vi "get_single_acq.vi"(8 "error in (no error)":errorcluster, 11 "dummy in":refnum<class "dummy.lvclass">) -> (0 "error out":errorcluster, 1 "trigger":bool[][](array[boolean]), 2 "raw data":i32[][][](array[numeric]), 3 "dummy out":refnum<class "dummy.lvclass">)   [LabVIEW 2019, in "dummy.lvlib" / "dummy.lvclass"]
uses:
  dummy.lvclass
  D:/github/TransientAbsorptionDAQ.lv/_camera/_camera.lvlibp/_cameraClass/_camera.lvclass
  _camera/_camera.lvlibp/_cameraClass/Read stage positions.vi
  _camera/_camera.lvlibp/_cameraClass/Read background.vi
  <vilib>/gmath/NI_Gmath.lvlib
  <vilib>/Analysis/NI_AALBase.lvlib
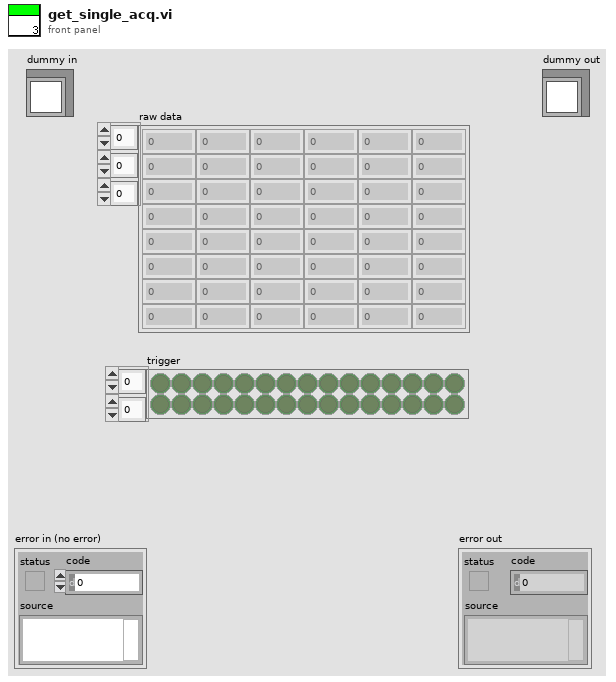
[diagram p1: front panel]
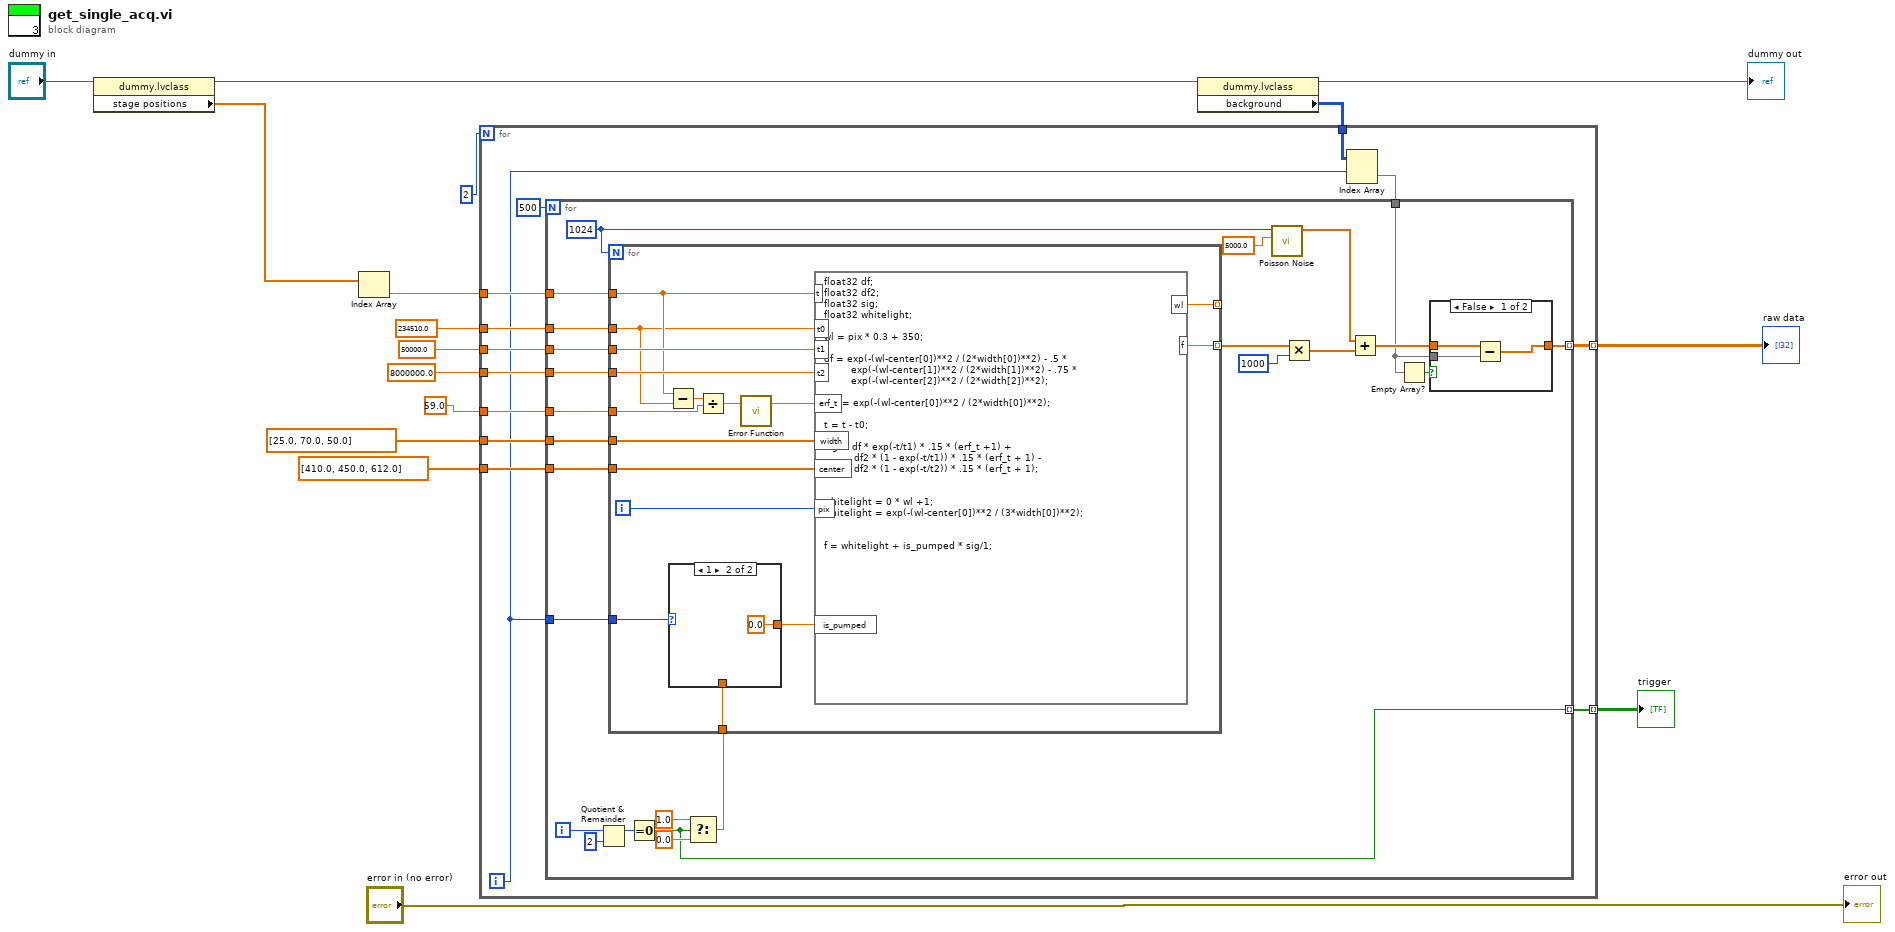
[diagram p0: block diagram]
diagram:
  n1 = property class="dummy.lvclass"(reference="dummy in") -> (reference out=w1:refnum<class "dummy.lvclass">, "stage positions"=w3:dbl[])  [unwired: 1 in, 1 out]
  n2 = Index Array(array=w3) -> (element=w5:dbl)  [unwired: 1 in]
  n3 = property class="dummy.lvclass"(reference=w1) -> (reference out=→"dummy out":refnum<class "dummy.lvclass">, "background"=w6:i32[][])  [unwired: 1 in, 1 out]
  n4 = for {
    N: 2 -> [_]
    tunnel: dbl[] [410.0, 450.0, 612.0] -> [w28]
    tunnel: dbl[] [25.0, 70.0, 50.0] -> [w27]
    tunnel: w5 -> [w26]
    tunnel: 234510.0 -> [w25]
    tunnel: 8000000.0 ("input variable") -> [w24]
    tunnel: 50000.0 ("input variable") -> [w23]
    tunnel: 59.0 ("y") -> [w22]
    tunnel: [w21] -> w9 mode=indexing
    tunnel: [w20] -> w8 mode=indexing
    tunnel: w6 -> [w19]
    i -> [w18]
    n5 = Index Array(array=w19, index (row)=w18) -> (element=w17:i32[])  [unwired: 1 in]
    n6 = for {
      N: 500 -> [_]
      tunnel: w28 -> [w54]
      tunnel: w27 -> [w53]
      tunnel: w26 -> [w52]
      tunnel: w25 -> [w51]
      tunnel: w24 -> [w50]
      tunnel: w23 -> [w49]
      tunnel: w22 -> [w48]
      tunnel: [w32] -> w21 mode=indexing
      tunnel: [w36] -> w20 mode=indexing
      tunnel: w18 -> [w35]
      tunnel: w17 -> [w30]
      i -> [w43]
      w40 = 1024
      n7 = Quotient & Remainder(x=w43, y=2) -> (x-y*floor(x/y)=w47:i32)  [unwired: 1 out]
      n8 = Equal To 0?(x=w47) -> (x = 0?=w36:bool)
      n9 = Select(t=1.0, s=w36, f=0.0) -> (s? t:f=w34:dbl)
      n10 = for {
        N: w40 -> [_]
        tunnel: w54 -> [w73]
        tunnel: w53 -> [w72]
        tunnel: w52 -> [w64]
        tunnel: w51 -> [w63]
        tunnel: w50 -> [w71]
        tunnel: w49 -> [w70]
        tunnel: w48 -> [w66]
        tunnel: [w62] -> w42 mode=indexing
        tunnel: [w65] -> _ mode=indexing
        tunnel: w35 -> [w61]
        tunnel: w34 -> [w59]
        i -> [w74]
        n11 = Subtract(x=w64, y=w63) -> (x-y=w68:dbl)
        n12 = case shown="1" w61 {
          tunnel: [w75 0.0 ("f")] -> w60
          tunnel: w59 -> [w75 _]
          frame 0, Default {
          }
          frame 1 {
          }
        }
        n13 = Divide(x=w68, y=w66) -> (x/y=w67:dbl)
        n14 = call <vilib>:"Error Function.vi"("x"=w67) -> ("erf(x)"=w69:dbl)  [unwired: 2 in]
        n15 = formula code="float32 df;\nfloat32 df2;\nfloat32 sig;\nfloat32 whitelight;\n\nwl = pix * 0.3 + 350;\n\ndf = exp(-(wl-center[0])**2 / (2*width[0])**2) - .5 *\n         exp(-(wl-center[1])**2 / (2*width[1])**2) - .75 * \n         exp(-(wl-center[2])**2 / (2*width[2])**2);\n\ndf2 = exp(-(wl-center[0])**2 / (2*width[0])**2);\n\nt = t - t0;\n\nsig = df * exp(-t/t1) * .15 * (erf_t +1) +\n          df2 * (1 - exp(-t/t1)) * .15 * (erf_t + 1) -\n          df2 * (1 - exp(-t/t2)) * .15 * (erf_t + 1);\n\n\nwhitelight = 0 * wl +1;\nwhitelight = exp(-(wl-center[0])**2 / (3*width[0])**2);\n\n\nf = whitelight + is_pumped * sig/1;"("pix"=w74, "center"=w73, "width"=w72, "t"=w64, "t0"=w63, "t1"=w70, "t2"=w71, "erf_t"=w69, "is_pumped"=w60) -> ("wl"=w65:dbl, "f"=w62:dbl)
      }
      n16 = call <vilib>:"Poisson Noise.vi"("mean"=5000.0, "samples"=w40) -> ("poisson noise"=w37:dbl[])  [unwired: 8 in, 1 out]
      n17 = Multiply(x=w42, y=1000) -> (x*y=w38:dbl[])
      n18 = Add(x=w37, y=w38) -> (x+y=w31:dbl[])
      n19 = Empty Array?(array=w30) -> (empty?=w33:bool)
      n20 = case shown="False" w33 {
        tunnel: [w55 w58] -> w32
        tunnel: w31 -> [w57 w58]
        tunnel: w30 -> [w56 _]
        frame False {
          n21 = Subtract(x=w57, y=w56) -> (x-y=w55:dbl[])
        }
        frame True {
        }
      }
    }
  }
  "raw data" <- w9
  "trigger" <- w8
  "error out" <- "error in (no error)"
